vi "VD-setRawMode.vi"(8 "error in (no error)":errorcluster, 10 "Free Running?":bool, 11 "VD-LV-LiteVNA in":refnum<class "VD-LV-LiteVNA.lvclass">) -> (0 "error out":errorcluster, 3 "VD-LV-LiteVNA out":refnum<class "VD-LV-LiteVNA.lvclass">)   [LabVIEW 2020, in "VD-LV-LiteVNA.lvclass"]
uses:
  VD-LV-LiteVNA.lvclass
  VD-action.ctl
  VD-LV-LiteVNA.lvclass/VD-LV-LiteVNA.ctl
  hardware-protocol/serial/HP-S-Serial.lvclass
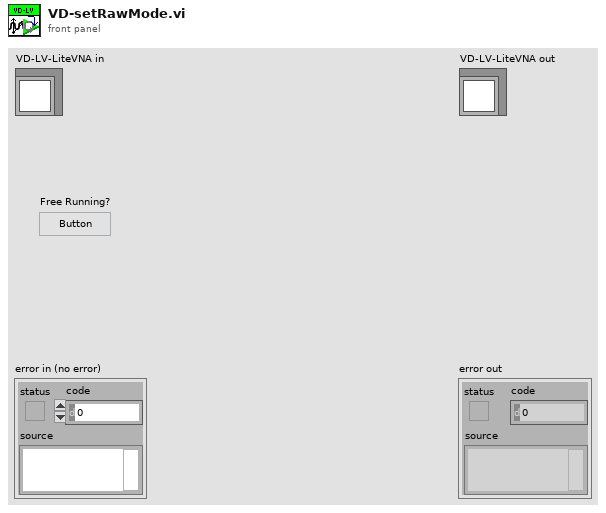
[diagram p1: front panel]
types:
  T1 = typedef "VD-LV-LiteVNA.lvclass/VD-action.ctl" = enum16{"checkCom", "SweepStartHz", "SweepStopHz", "SweepPoints", "valuesPerFrequency", "RawSamplesMode", "ValuesFIFO", "deviceVariant", "protocolVersion", "hardwareRevision", "firmwareMajor", "firmwareMinor"}
  T2 = typedef "HP-S-Serial.lvclass/HP-S-data.ctl" = u8[]
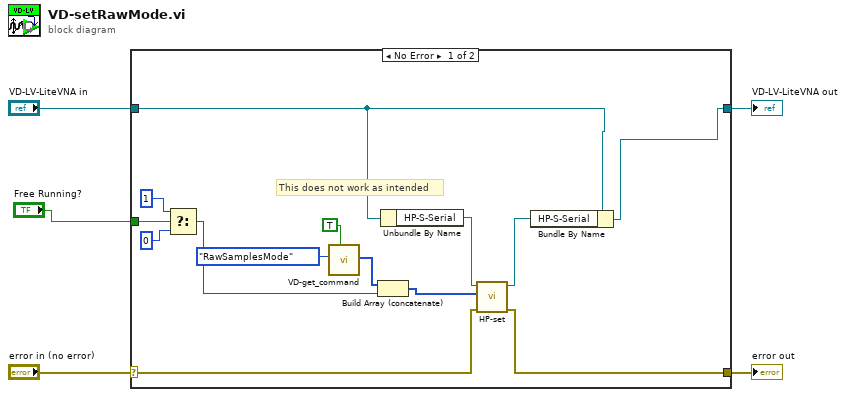
[diagram p0: block diagram]
diagram:
  n1 = case shown="No Error" "error in (no error)" {
    selector: "error in (no error)" -> [w7 w21]
    tunnel: [w6 w21] -> w4
    tunnel: [w13 w20] -> w2
    tunnel: "VD-LV-LiteVNA in" -> [w14 w20]
    tunnel: "Free Running?" -> [w12 _]
    frame No Error {
      # "This does not work as intended"
      n2 = Select(t=u8 1 ("8bit"), s=w12, f=u8 0 ("8bit")) -> (s? t:f=w9:u8)
      n3 = call "VD-get_command.vi"("Write?"=TRUE, "action"=VD-action."RawSamplesMode") -> ("Command"=w17:T2)  [unwired: 9 in]
      n4 = Build Array (concatenate)(w17, w9) -> (w8:T2)
      n5 = Unbundle By Name(w14) -> ("HP-S-Serial"=w19:refnum<class "HP-S-Serial.lvclass">)
      n6 = call-dynamic "HP-set.vi"("error in (no error)"=w7, "write buffer"=w8, "HP-S-Serial in"=w19) -> ("error out"=w6:errorcluster, "HP-S-Serial out"=w18:refnum<class "HP-S-Serial.lvclass">)  [unwired: 7 in]
      n7 = Bundle By Name(cluster=w14, "HP-S-Serial"=w18) -> (w13:refnum<class "VD-LV-LiteVNA.lvclass">)
    }
    frame Error {
    }
  }
  "error out" <- w4
  "VD-LV-LiteVNA out" <- w2
